vi "mqttCmdAcknowledge.vi"(0 "_mqtt in":refnum<class "mqttCmdSubscribe.lvclass">, 11 "error in (no error)":errorcluster) -> (4 "_mqtt out":refnum<class "mqttCmdSubscribe.lvclass">, 8 "notification":T1, 15 "error out":errorcluster)   [LabVIEW 2017, in "mqttCmdSubscribe.lvclass"]
uses:
  mqttCmdSubscribe.lvclass
  C:/Users/claessen/Documents/mqtt-LabVIEW/src/class/mqtt/mqttCmd/mqttCmd.lvclass
  mqttTypedef/mqttRXdataCluster.ctl
  mqttTypedef/mqttFixedHeaderResponse.ctl
  mqttTypedef/mqttQOSlevel.ctl
  mqttTypedef/mqttMessageType.ctl
  mqttCmd.lvclass/mqttCmd.ctl
  mqttCmdSubscribe.lvclass/mqttCmdSubscribe.ctl
  mqttCmd.lvclass
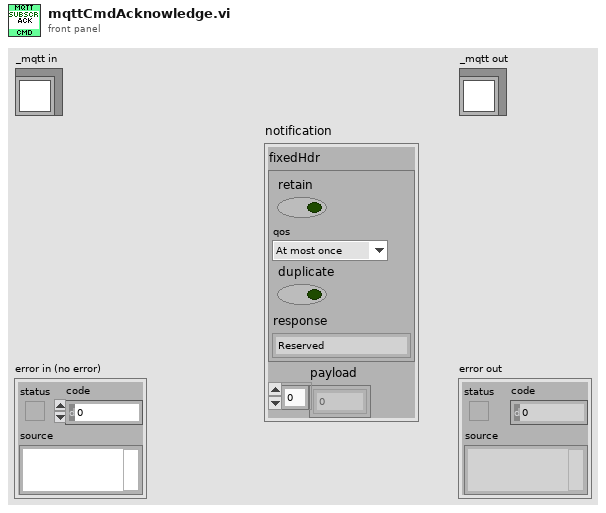
[diagram p1: front panel]
types:
  T1 = typedef "mqttRXdataCluster.ctl" = cluster{"fixedHdr":T2, "payload":u8[]}
  T2 = typedef "mqttFixedHeaderResponse.ctl" = cluster{"retain":bool, "qos":T3, "duplicate":bool, "response":T4}
  T3 = typedef "mqttQOSlevel.ctl" = enum8{"At most once", "At least once", "Exactly once", "Reserved"}
  T4 = typedef "mqttMessageType.ctl" = enum32{"Reserved", "CONNECT", "CONNACK", "PUBLISH", "PUBACK", "PUBREC", "PUBREL", "PUBCOMP", "SUBSCRIBE", "SUBACK", "UNSUBSCRIBE", "UNSUBACK", "PINGREQ", "PINGRESP", "DISCONNECT", "Reserved2"}
  T5 = typedef "mqttSubscribeCluster.ctl" = cluster{"Topic":string, "QoS":T3}
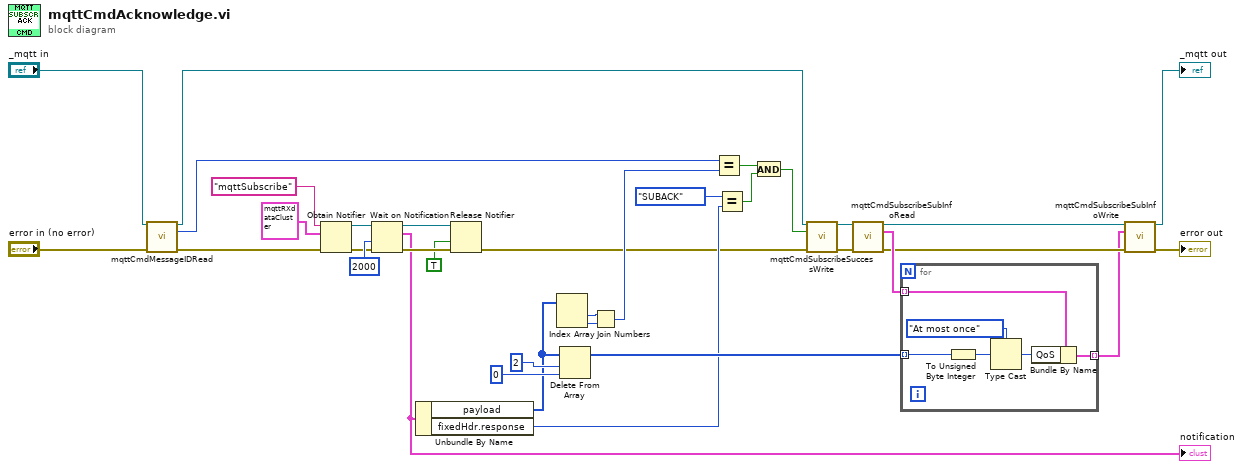
[diagram p0: block diagram]
diagram:
  n1 = call "mqttCmdMessageIDRead.vi"("mqttBrokerCommand in"="_mqtt in", "error in (no error)"="error in (no error)") -> ("mqttBrokerCommand out"=w13:refnum<class "mqttCmdSubscribe.lvclass">, "messageID"=w12:u16, "error out"=w15:errorcluster)  [unwired: 11 in]
  n2 = Obtain Notifier(name (unnamed)="mqttSubscribe", notification data type=T1 {"fixedHdr"={"retain"=FALSE, "qos"=enum."At most once", "duplicate"=FALSE, "response"=enum."Reserved"}, "payload"=[]} ("notification"), error in (no error)=w15) -> (notifier out=w21:refnum<notifier>, error out=w18:errorcluster)  [unwired: 1 in, 1 out]
  n3 = Wait on Notification(notifier=w21, timeout in ms (-1)=2000, error in (no error)=w18) -> (notifier out=w27:refnum<notifier>, notification=w10:T1, error out=w26:errorcluster)  [unwired: 1 in, 1 out]
  "notification" <- w10
  n4 = Unbundle By Name(w10) -> ("payload"=w28:u8[], "fixedHdr.response"=w11:T4)
  n5 = Release Notifier(notifier=w27, force destroy? (F)=TRUE, error in (no error)=w26) -> (error out=w9:errorcluster)  [unwired: 2 out]
  n6 = Index Array(array=w28) -> (element #1=w24:u8, element #2=w23:u8)  [unwired: 2 in]
  n7 = Delete From Array(array=w28, length=2, index=0) -> (array with subset deleted=w35:u8[])  [unwired: 1 out]
  n8 = Join Numbers(hi=w24, lo=w23) -> ((hi.lo)=w34:u16)
  n9 = Equal?(x=w12, y=w34) -> (x = y?=w31:bool)
  n10 = Equal?(x=mqttMessageType."SUBACK", y=w11) -> (x = y?=w32:bool)
  n11 = And(x=w31, y=w32) -> (x .and. y?=w17:bool)
  n12 = call "mqttCmdSubscribeSuccessWrite.vi"("mqttBrokerCommand in"=w13, "success"=w17, "error in (no error)"=w9) -> ("mqttBrokerCommand out"=w7:refnum<class "mqttCmdSubscribe.lvclass">, "error out"=w8:errorcluster)  [unwired: 11 in]
  n13 = call "mqttCmdSubscribeSubInfoRead.vi"("mqttSubscribe in"=w7, "error in (no error)"=w8) -> ("mqttSubscribe out"=w3:refnum<class "mqttCmdSubscribe.lvclass">, "subscriptionInfo"=w6:T5[], "error out"=w5:errorcluster)  [unwired: 11 in]
  n14 = for {
    tunnel: w35 -> [w40] mode=indexing
    tunnel: w6 -> [w38] mode=indexing
    tunnel: [w36] -> w4 mode=indexing
    n15 = To Unsigned Byte Integer(number=w40) -> (unsigned 8bit integer=w41:u8)
    n16 = Type Cast(type=mqttQOSlevel."At most once" ("fixedHdr.qos"), x=w41) -> (*(type *) &x=w37:T3)
    n17 = Bundle By Name(cluster=w38, "QoS"=w37) -> (w36:T5)
  }
  n18 = call "mqttCmdSubscribeSubInfoWrite.vi"("mqttSubscribe in"=w3, "subscriptionInfo"=w4, "error in (no error)"=w5) -> ("mqttSubscribe out"=→"_mqtt out":refnum<class "mqttCmdSubscribe.lvclass">, "error out"=→"error out":errorcluster)  [unwired: 11 in]
